vi "Read Actor List.vi"(8 "error in (no error)":errorcluster, 11 "CS++StartActor in":refnum<class "CS++StartActor.lvclass">) -> (0 "error out":errorcluster, 3 "CS++StartActor out":refnum<class "CS++StartActor.lvclass">)   [LabVIEW 2013, in "CS++StartActor.lvlib" / "CS++StartActor.lvclass"]
doc: "Read Actor List from DB Connection."
uses:
  CS++StartActor.lvclass
  CS++BaseActor/CS++BaseActor.lvclass/CS++BaseActor.ctl
  Classes/CS++BaseClasses/Factory/CS++Factory.lvclass
  CS++StartActor.lvclass/CS++StartActor.ctl
  Libraries/Base/CS++Base.lvlib
  CS++BaseActor/CS++BaseActor.lvclass
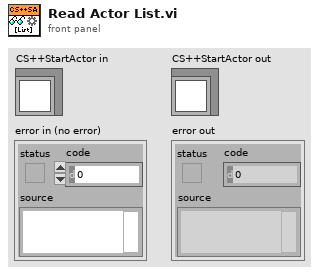
[diagram p1: front panel]
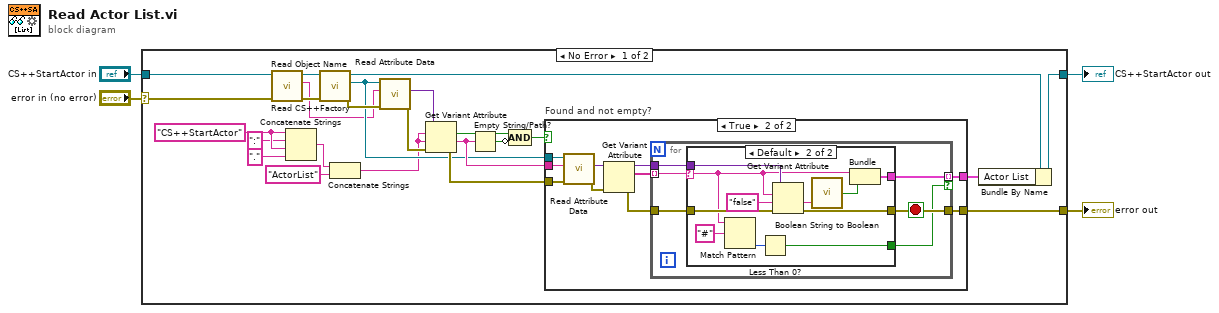
[diagram p0: block diagram]
diagram:
  n1 = case shown="No Error" "error in (no error)" {
    selector: "error in (no error)" -> [w8 w58]
    tunnel: [w11 w58] -> w3
    tunnel: [w13 w57] -> w1
    tunnel: "CS++StartActor in" -> [w10 w57]
    frame No Error {
      w23 = "CS++StartActor"
      n2 = call "Read Object Name.vi"("error in (no error)"=w8, "CS++BaseActor in"=w10) -> ("error out"=w7:errorcluster, "Object Name"=w6:string, "CS++BaseActor out"=w9:refnum<class "CS++StartActor.lvclass">)  [unwired: 7 in]
      n3 = Concatenate Strings(w23, ":" ("string"), w23, "." ("string")) -> (w20:string)
      n4 = call "Read CS++Factory.vi"("error in (no error)"=w7, "CS++BaseActor in"=w9) -> ("error out"=w18:errorcluster, "CS++Factory"=w15:refnum<class "CS++Factory.lvclass">, "CS++BaseActor out"=w14:refnum<class "CS++StartActor.lvclass">)  [unwired: 7 in]
      n5 = Concatenate Strings(w20, "ActorList" ("string")) -> (w5:string)
      n6 = call-dynamic "Read Attribute Data.vi"("error in (no error)"=w18, "Object Name"=w6, "CS++Factory in"=w15) -> ("error out"=w17:errorcluster, "Attribute Data"=w19:variant)  [unwired: 6 in, 1 out]
      n7 = Get Variant Attribute(Variant=w19, name=w5, default value (empty Variant)=w5, error in=w17) -> (found=w28:bool, value=w25:string, error out=w26:errorcluster)  [unwired: 1 out]
      n8 = Empty String/Path?(string/path=w25) -> (empty?=w27:bool)
      n9 = Compound Arithmetic op=AND(w28, invert w27) -> (w24:bool)
      n10 = case "Found and not empty?" shown="True" w24 {
        tunnel: [_ w34] -> w12
        tunnel: [w29 w33] -> w11
        tunnel: w15 -> [_ w32]
        tunnel: w26 -> [w29 w31]
        tunnel: w25 -> [_ w30]
        frame False {
        }
        frame True {
          n11 = call-dynamic "Read Attribute Data.vi"("error in (no error)"=w31, "Object Name"=w30, "CS++Factory in"=w32) -> ("error out"=w36:errorcluster, "Attribute Data"=w35:variant)  [unwired: 6 in, 1 out]
          n12 = Get Variant Attribute(Variant=w35, error in=w36) -> (duplicate Variant=w38:variant, names=w37:string[], error out=w39:errorcluster)  [unwired: 2 in, 1 out]
          n13 = for {
            tunnel: w37 -> [w40] mode=indexing
            tunnel: [w42] -> w34 mode=indexing if=w41
            tunnel: w38 -> [w45]
            tunnel: w39 -> [w44]
            tunnel: [w43] -> w33
            stop <- w43 stop-if-true
            n14 = case shown="Default" w40 {
              selector: w40 -> [_ w46]
              tunnel: w45 -> [_ w56]
              tunnel: w44 -> [_ w55]
              tunnel: [_ w54] -> w43
              tunnel: [_ w50] -> w42
              tunnel: [_ w47] -> w41
              frame "CS++ObjectName" {
              }
              frame Default {
                n15 = Match Pattern(string=w46, regular expression="#") -> (offset past match=w48:i32)  [unwired: 1 in, 3 out]
                n16 = Less Than 0?(x=w48) -> (x < 0?=w47:bool)
                n17 = Get Variant Attribute(Variant=w56, name=w46, default value (empty Variant)="false" ("string"), error in=w55) -> (value=w52:string, error out=w54:errorcluster)  [unwired: 2 out]
                n18 = call "Boolean String to Boolean.vi"("T/F String"=w52) -> ("Value"=w51:bool)
                n19 = Bundle(w46, "Value"=w51) -> (w50:cluster{string, "Value":bool})  [unwired: 1 in]
              }
            }
          }
        }
      }
      n20 = Bundle By Name(cluster=w14, "Actor List"=w12) -> (w13:refnum<class "CS++StartActor.lvclass">)
    }
    frame Error {
    }
  }
  "error out" <- w3
  "CS++StartActor out" <- w1
